vi "LKIF_SetPanelLock.vi"(8 "error in (no error)":errorcluster {"code" format="%x"}, 11 "IsLock":bool) -> (0 "error out":errorcluster {"code" format="%x"})   [LabVIEW 2024, in "Keyence LK-G3000.lvlib"]
uses:
  Keyence LK-G3000.lvlib
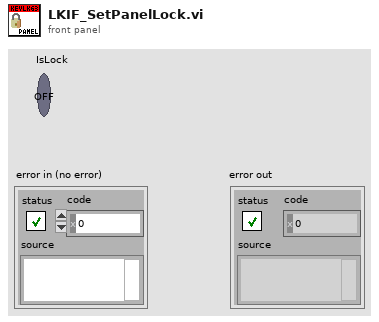
[diagram p1: front panel]
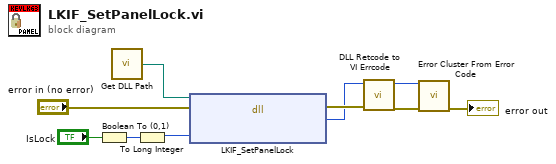
[diagram p0: block diagram]
diagram:
  n1 = Boolean To (0,1)(Boolean="IsLock") -> (0, 1=w6:i16)
  n2 = call "Get DLL Path.vi"() -> ("DLL Path"=w1:path)  [unwired: 1 in]
  n3 = To Long Integer(number=w6) -> (32bit integer=w4:i32)
  n4 = dll-call lib="C:/Program Files/National Instruments/LabVIEW 2011/instr.lib/Keyence LK-G3000/LkIF.dll" fn="LKIF_SetPanelLock"(path in=w1, error in="error in (no error)", "IsLock"=w4) -> (error out=w3:errorcluster, "RC"=w2:i32)  [unwired: 2 in, 1 out]
  n5 = call "DLL Retcode to VI Errcode.vi"("error in (no error)"=w3, "DLL Retcode"=w2) -> ("error out"=w10:errorcluster, "VI Errcode"=w9:i32)  [unwired: 8 in]
  n6 = call <vilib>:"Error Cluster From Error Code.vi"("error in (no error)"=w10, "error code (0)"=w9) -> ("error out"=→"error out":errorcluster)  [unwired: 7 in]
